vi "Write Size.vi"(8 "error in (no error)":errorcluster, 10 "Size":T1, 11 "IOName.lvclass in":refnum<class "IOName.lvclass">) -> (0 "error out":errorcluster, 3 "IOName.lvclass out":refnum<class "IOName.lvclass">)   [LabVIEW 2015, in "IOName.lvclass"]
uses:
  IOName.lvclass
  <vilib>/Utility/miscctls.llb/LVBoundsTypeDef.ctl
  IOName.lvclass/IOName.ctl
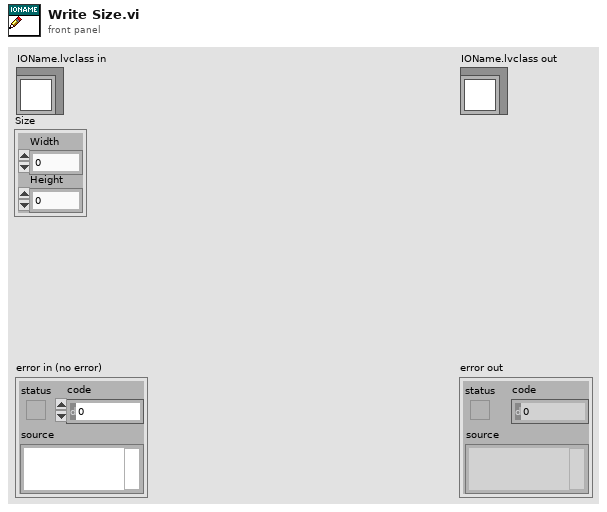
[diagram p1: front panel]
types:
  T1 = typedef "LVBoundsTypeDef.ctl" = cluster{"Width":u32, "Height":u32}
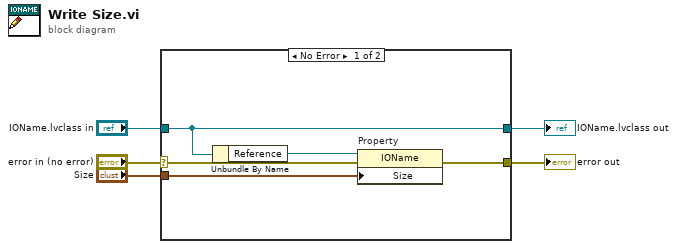
[diagram p0: block diagram]
diagram:
  n1 = case shown="No Error" "error in (no error)" {
    selector: "error in (no error)" -> [w6 w12]
    tunnel: [w10 w12] -> w4
    tunnel: [w8 w11] -> w2
    tunnel: "IOName.lvclass in" -> [w8 w11]
    tunnel: "Size" -> [w9 _]
    frame No Error {
      n2 = Unbundle By Name(w8) -> ("Reference"=w7:refnum<vi>)
      n3 = property on="Property" class="IOName"(reference=w7, error in=w6, "Size"=w9) -> (error out=w10:errorcluster)  [unwired: 1 out]
    }
    frame Error {
    }
  }
  "error out" <- w4
  "IOName.lvclass out" <- w2
